vi "Set Connection Properties.vi"(8 "error in (no error)":errorcluster, 10 "AutoSelect":T2, 11 "Device Item Ref in":T1 format="%.0x") -> (0 "error out":errorcluster, 3 "Item Ref out":T1 format="%.0x")   [LabVIEW 2019, in "NI Synchronization System Explorer.lvlib"]
uses:
  NI Synchronization System Explorer.lvlib
  Shared/Connection Settings.ctl
  Shared/Mode.ctl
  Shared/External Pin.ctl
  Shared/Routes.ctl
  Shared/Route.ctl
  <vilib>/NI VeriStand/Custom Device API/Custom Device Item Ref.ctl
  Shared/Constants.vi
  <vilib>/NI VeriStand/Custom Device API/Set Item Property (U16).vi
  <vilib>/NI VeriStand/Custom Device API/Set Item Property (Boolean).vi
  Shared/NI Synchronization Shared.lvlib
  <vilib>/NI VeriStand/Custom Device API/Custom Device API.lvlib
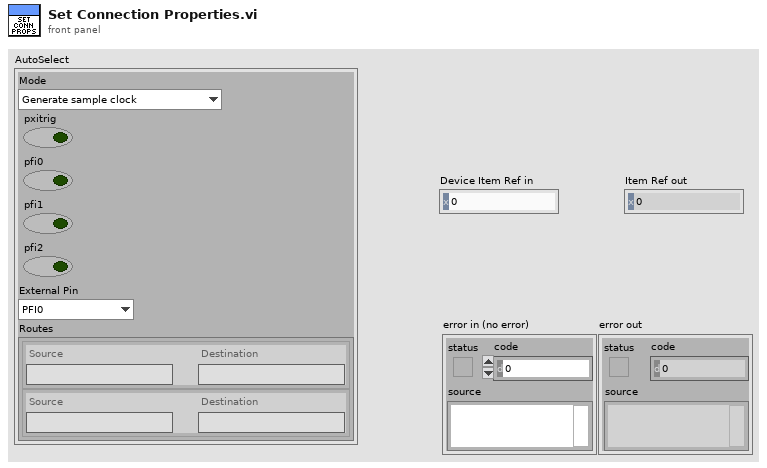
[diagram p1: front panel]
types:
  T1 = typedef "Custom Device API.lvlib/Custom Device Item Ref.ctl" = u64
  T2 = typedef "NI Synchronization Shared.lvlib/Connection Settings.ctl" = cluster{"Mode":T3, "pxitrig":bool, "pfi0":bool, "pfi1":bool, "pfi2":bool, "External Pin":T4, "Routes":T5}
  T3 = typedef "NI Synchronization Shared.lvlib/Mode.ctl" = enum16{"Generate sample clock", "Route sample clock out of chassis", "Route sample clock into chassis", "Custom routes"}
  T4 = typedef "NI Synchronization Shared.lvlib/External Pin.ctl" = enum16{"PFI0", "PFI1", "PFI2"}
  T5 = typedef "NI Synchronization Shared.lvlib/Routes.ctl" = T6[]
  T6 = typedef "NI Synchronization Shared.lvlib/Route.ctl" = cluster{"Source":string, "Destination":string}
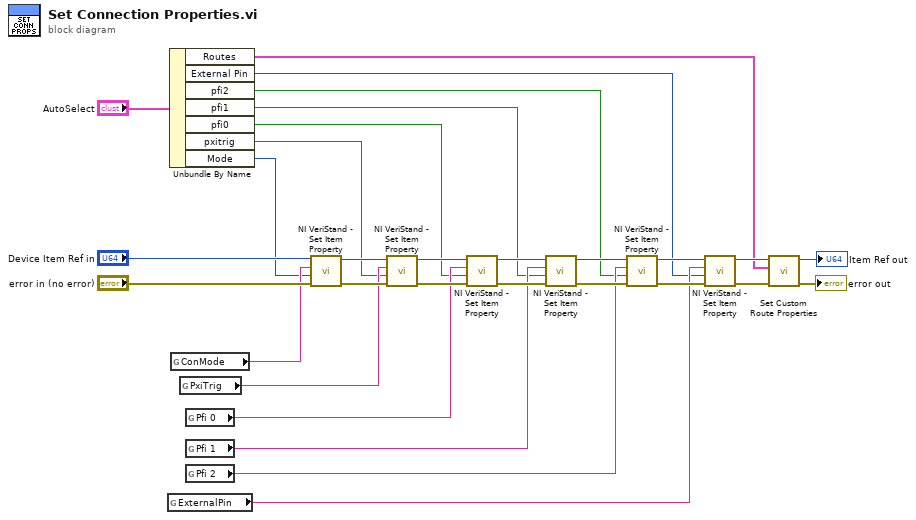
[diagram p0: block diagram]
diagram:
  n1 = global read "Constants.vi" "ExternalPin"() -> (w13:string)
  n2 = Unbundle By Name("AutoSelect") -> ("Routes"=w3:T5, "External Pin"=w2:T4, "pfi2"=w4:bool, "pfi1"=w5:bool, "pfi0"=w6:bool, "pxitrig"=w7:bool, "Mode"=w1:T3)
  n3 = global read "Constants.vi" "ConMode"() -> (w28:string)
  n4 = global read "Constants.vi" "PxiTrig"() -> (w25:string)
  n5 = global read "Constants.vi" "Pfi 0"() -> (w22:string)
  n6 = global read "Constants.vi" "Pfi 1"() -> (w19:string)
  n7 = global read "Constants.vi" "Pfi 2"() -> (w16:string)
  n8 = call-poly <vilib>:"NI VeriStand - Set Item Property.vi"("error in (no error)"="error in (no error)", "Value"=w1, "Property Name"=w28, "Item Ref in"="Device Item Ref in") -> ("error out"=w26:errorcluster, "Item Ref out"=w27:T1)  [unwired: 5 in, 1 out]
  n9 = call-poly <vilib>:"NI VeriStand - Set Item Property.vi"("error in (no error)"=w26, "Value"=w7, "Property Name"=w25, "Item Ref in"=w27) -> ("error out"=w23:errorcluster, "Item Ref out"=w24:T1)  [unwired: 5 in, 1 out]
  n10 = call-poly <vilib>:"NI VeriStand - Set Item Property.vi"("error in (no error)"=w23, "Value"=w6, "Property Name"=w22, "Item Ref in"=w24) -> ("error out"=w20:errorcluster, "Item Ref out"=w21:T1)  [unwired: 5 in, 1 out]
  n11 = call-poly <vilib>:"NI VeriStand - Set Item Property.vi"("error in (no error)"=w20, "Value"=w5, "Property Name"=w19, "Item Ref in"=w21) -> ("error out"=w17:errorcluster, "Item Ref out"=w18:T1)  [unwired: 5 in, 1 out]
  n12 = call-poly <vilib>:"NI VeriStand - Set Item Property.vi"("error in (no error)"=w17, "Value"=w4, "Property Name"=w16, "Item Ref in"=w18) -> ("error out"=w15:errorcluster, "Item Ref out"=w14:T1)  [unwired: 5 in, 1 out]
  n13 = call-poly <vilib>:"NI VeriStand - Set Item Property.vi"("error in (no error)"=w15, "Value"=w2, "Property Name"=w13, "Item Ref in"=w14) -> ("error out"=w12:errorcluster, "Item Ref out"=w11:T1)  [unwired: 5 in, 1 out]
  n14 = call "Set Custom Route Properties.vi"("error in (no error)"=w12, "Routes"=w3, "Item Ref in"=w11) -> ("error out"=→"error out":errorcluster, "Item Ref out"=→"Item Ref out":T1)  [unwired: 7 in]
